vi "[Example] Send Message and Image to Slack Channel.vi"() -> ()   [LabVIEW 2018]
uses:
  Slack API/Slack API.lvlib
panel:
  in  "image filepath":path
  in  "API token":string
  in  "Channel":string
  in  "message":string
  # "Slack Workspace"
  # "Getting Started\n\nSlack\n1. Create or find your Slack workspace (https://slack.com/get-started)\n2. Create a bot and save the bot's API token somewhere (https://api.slack.com/bot-users).  Use this API token in this VI.\n3. Create a new channel in your Slack workspace if necessary.  In this VI, specify the Slack channel you want this VI to send a message or image.\n\nPython\n1. Install slackclient v2.0.0 using the \"pip install slackclient=2.0.0\" command."
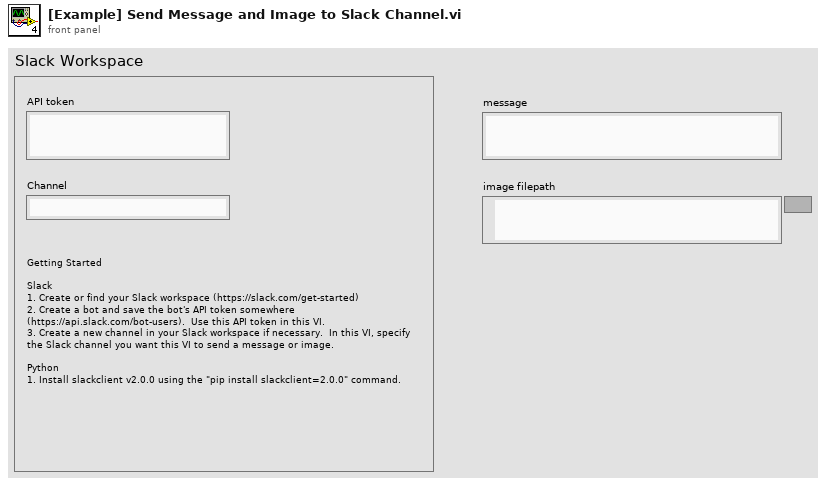
[diagram p1: front panel]
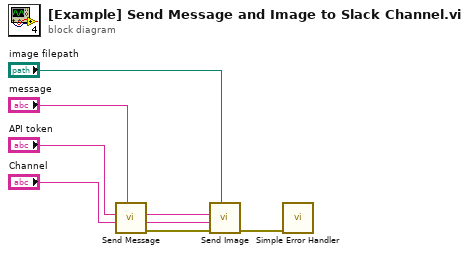
[diagram p0: block diagram]
diagram:
  n1 = call "Send Message.vi"("message"="message", "slack channel"="Channel", "slack API token"="API token") -> ("error out"=w3:errorcluster, "slack channel dup"=w4:string, "slack API token dup"=w5:string)  [unwired: 6 in]
  n2 = call "Send Image.vi"("image filepath"="image filepath", "error in (no error)"=w3, "slack channel"=w4, "slack API token"=w5) -> ("error out"=w1:errorcluster)  [unwired: 5 in, 2 out]
  n3 = call <vilib>:"Simple Error Handler.vi"("error in (no error)"=w1) -> ()  [unwired: 4 in, 5 out]
